vi "unregister_swabian_events.vi"(8 "error in (no error)":errorcluster, 11 "references":T1) -> (0 "error out":errorcluster)   [LabVIEW 2018]
uses:
  swabian_event_refs.ctl
  update_chart_tdef.ctl
  channel_data_tdef.ctl
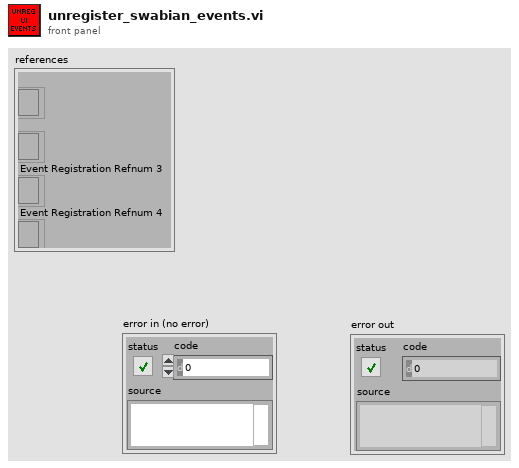
[diagram p1: front panel]
types:
  T1 = typedef "swabian_event_refs.ctl" = cluster{"event registration refnum":refnum<event-registration>, "Event Registration Refnum 2":refnum<event-registration>, "Event Registration Refnum 3":refnum<event-registration>, "Event Registration Refnum 4":refnum<event-registration>}
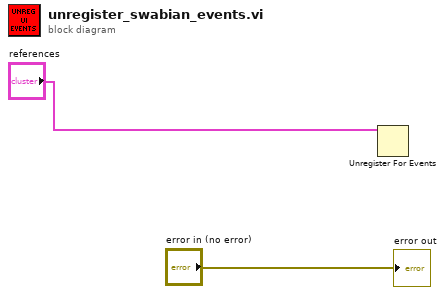
[diagram p0: block diagram]
diagram:
  n1 = Unregister For Events(event registration refnum="references") -> ()  [unwired: 1 in, 1 out]
  "error out" <- "error in (no error)"
